vi "GOMDBTS2048 two devices sample.vi"() -> ()   [LabVIEW 2009]
panel:
  out "XY Graph 2":cluster{i32, dbl}[](graph)
  out "XY Graph":cluster{i32, dbl}[](graph)
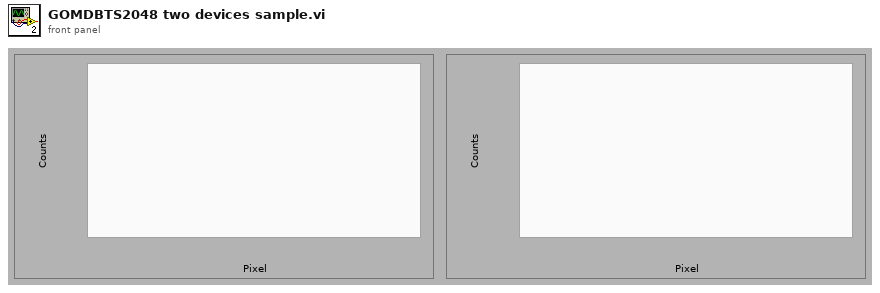
[diagram p1: front panel]
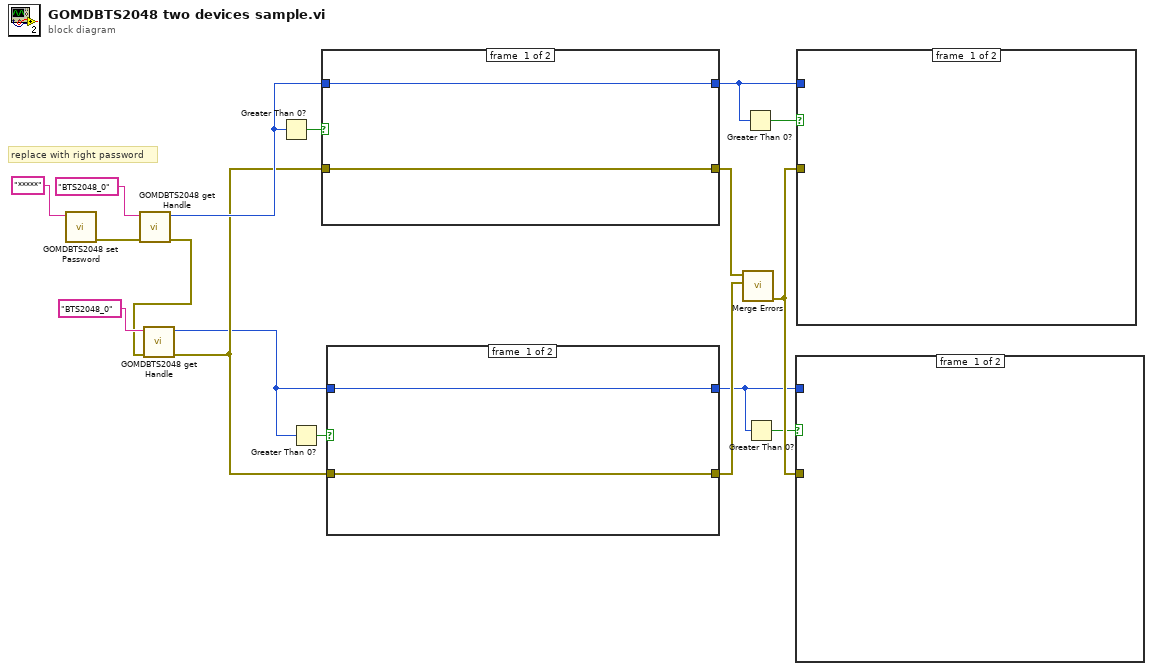
[diagram p0: block diagram]
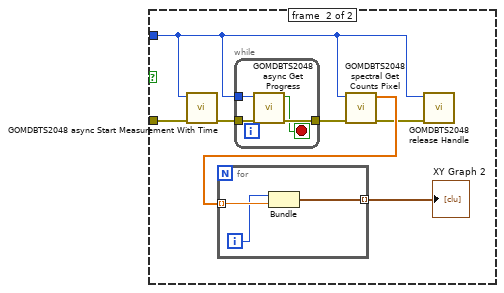
[diagram p2: hidden frame]
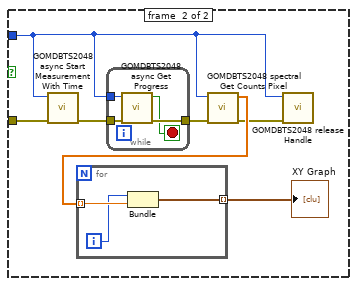
[diagram p3: hidden frame]
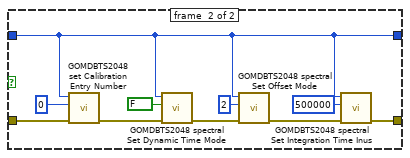
[diagram p4: hidden frame]
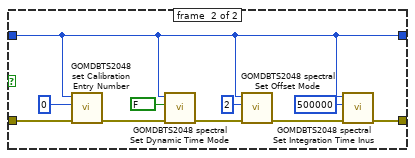
[diagram p5: hidden frame]
diagram:
  # "replace with right password"
  n1 = call <userlib>:"GOMDBTS2048 set Password.vi"("value"="*****" ("deviceName")) -> ("error out"=w1:errorcluster)  [unwired: 9 in, 1 out]
  n2 = call <userlib>:"GOMDBTS2048 get Handle.vi"("error in (no error)"=w1, "device"="BTS2048_0" ("deviceName")) -> ("error out"=w7:errorcluster, "handle"=w14:i32)  [unwired: 7 in, 1 out]
  n3 = call <userlib>:"GOMDBTS2048 get Handle.vi"("error in (no error)"=w7, "device"="BTS2048_0" ("deviceName")) -> ("error out"=w13:errorcluster, "handle"=w12:i32)  [unwired: 7 in, 1 out]
  n4 = Greater Than 0?(x=w14) -> (x > 0?=w11:bool)
  n5 = Greater Than 0?(x=w12) -> (x > 0?=w10:bool)
  n6 = case shown="True" w11 {
    tunnel: w14 -> [w18 w20]
    tunnel: w13 -> [w19 w29]
    tunnel: [w19 w25] -> w9
    tunnel: [w18 w20] -> w6
    frame #0 {
    }
    frame #1 {
      n7 = call <userlib>:"GOMDBTS2048 set Calibration Entry Number.vi"("error in (no error)"=w29, "calibrationEntryNumber"=0, "handle"=w20) -> ("error out"=w28:errorcluster)  [unwired: 7 in, 1 out]
      n8 = call <userlib>:"GOMDBTS2048 spectral Set Dynamic Time Mode.vi"("error in (no error)"=w28, "value"=FALSE, "handle"=w20) -> ("error out"=w27:errorcluster)  [unwired: 7 in, 1 out]
      n9 = call <userlib>:"GOMDBTS2048 spectral Set Offset Mode.vi"("error in (no error)"=w27, "value"=2, "handle"=w20) -> ("error out"=w26:errorcluster)  [unwired: 7 in, 1 out]
      n10 = call <userlib>:"GOMDBTS2048 spectral Set Integration Time Inus.vi"("error in (no error)"=w26, "timeInus"=500000, "handle"=w20) -> ("error out"=w25:errorcluster)  [unwired: 7 in, 1 out]
    }
  }
  n11 = case shown="True" w10 {
    tunnel: w13 -> [w31 w41]
    tunnel: w12 -> [w30 w32]
    tunnel: [w31 w37] -> w8
    tunnel: [w30 w32] -> w4
    frame #0 {
    }
    frame #1 {
      n12 = call <userlib>:"GOMDBTS2048 set Calibration Entry Number.vi"("error in (no error)"=w41, "calibrationEntryNumber"=0, "handle"=w32) -> ("error out"=w40:errorcluster)  [unwired: 7 in, 1 out]
      n13 = call <userlib>:"GOMDBTS2048 spectral Set Dynamic Time Mode.vi"("error in (no error)"=w40, "value"=FALSE, "handle"=w32) -> ("error out"=w39:errorcluster)  [unwired: 7 in, 1 out]
      n14 = call <userlib>:"GOMDBTS2048 spectral Set Offset Mode.vi"("error in (no error)"=w39, "value"=2, "handle"=w32) -> ("error out"=w38:errorcluster)  [unwired: 7 in, 1 out]
      n15 = call <userlib>:"GOMDBTS2048 spectral Set Integration Time Inus.vi"("error in (no error)"=w38, "timeInus"=500000, "handle"=w32) -> ("error out"=w37:errorcluster)  [unwired: 7 in, 1 out]
    }
  }
  n16 = call <vilib>:"Merge Errors.vi"("error in 2 (no error)"=w8, "error in 1 (no error)"=w9) -> ("error out"=w5:errorcluster)  [unwired: 5 in]
  n17 = Greater Than 0?(x=w6) -> (x > 0?=w2:bool)
  n18 = Greater Than 0?(x=w4) -> (x > 0?=w3:bool)
  n19 = case shown="True" w3 {
    tunnel: w5 -> [_ w45]
    tunnel: w4 -> [_ w42]
    frame #0 {
    }
    frame #1 {
      n20 = call <userlib>:"GOMDBTS2048 async Start Measurement With Time.vi"("error in (no error)"=w45, "handle"=w42) -> ("error out"=w44:errorcluster)  [unwired: 7 in, 2 out]
      n21 = while {
        tunnel: w44 -> [w52]
        tunnel: [w51] -> w43
        tunnel: w42 -> [w49]
        stop <- w50 stop-if-true
        n22 = call <userlib>:"GOMDBTS2048 async Get Progress.vi"("error in (no error)"=w52, "handle"=w49) -> ("error out"=w51:errorcluster, "finished"=w50:bool)  [unwired: 6 in, 2 out]
      }
      n23 = call <userlib>:"GOMDBTS2048 spectral Get Counts Pixel.vi"("error in (no error)"=w43, "handle"=w42) -> ("error out"=w46:errorcluster, "counts"=w47:dbl[])  [unwired: 7 in, 1 out]
      n24 = for {
        tunnel: w47 -> [w55] mode=indexing
        tunnel: [w53] -> w48 mode=indexing
        i -> [w54]
        n25 = Bundle(w54, w55) -> (w53:cluster{i32, dbl})  [unwired: 1 in]
      }
      "XY Graph 2" <- w48
      n26 = call <userlib>:"GOMDBTS2048 release Handle.vi"("error in (no error)"=w46, "handle"=w42) -> ()  [unwired: 8 in, 2 out]
    }
  }
  n27 = case shown="True" w2 {
    tunnel: w6 -> [_ w58]
    tunnel: w5 -> [_ w59]
    frame #0 {
    }
    frame #1 {
      n28 = call <userlib>:"GOMDBTS2048 async Start Measurement With Time.vi"("error in (no error)"=w59, "handle"=w58) -> ("error out"=w57:errorcluster)  [unwired: 7 in, 2 out]
      n29 = while {
        tunnel: w58 -> [w66]
        tunnel: w57 -> [w65]
        tunnel: [w64] -> w56
        stop <- w63 stop-if-true
        n30 = call <userlib>:"GOMDBTS2048 async Get Progress.vi"("error in (no error)"=w65, "handle"=w66) -> ("error out"=w64:errorcluster, "finished"=w63:bool)  [unwired: 6 in, 2 out]
      }
      n31 = call <userlib>:"GOMDBTS2048 spectral Get Counts Pixel.vi"("error in (no error)"=w56, "handle"=w58) -> ("error out"=w60:errorcluster, "counts"=w61:dbl[])  [unwired: 7 in, 1 out]
      n32 = for {
        tunnel: w61 -> [w69] mode=indexing
        tunnel: [w67] -> w62 mode=indexing
        i -> [w68]
        n33 = Bundle(w68, w69) -> (w67:cluster{i32, dbl})  [unwired: 1 in]
      }
      "XY Graph" <- w62
      n34 = call <userlib>:"GOMDBTS2048 release Handle.vi"("error in (no error)"=w60, "handle"=w58) -> ()  [unwired: 8 in, 2 out]
    }
  }
